vi "Actor Core.vi"(8 "error in":errorcluster, 11 "BNT_DSCXYGraph in":refnum<class "BNT_DSCXYGraph.lvclass">) -> (0 "error out":errorcluster, 3 "Actor out":refnum<class "Actor.lvclass">)   [LabVIEW 2017, in "BNT_DSCXYGraph.lvlib" / "BNT_DSCXYGraph.lvclass"]
doc: "(<B>Filename</B>: Actor Framework.lvlib:Actor.lvclass:Actor Core.vi)\n\nReceives messages to the actor, reacts to them, and initiates any error handling that may shut the actor down.\n\nDescendant classes may override this VI to append parallel tasks for the actor to complete while it handles messages. Overrides use the Call Parent Method node."
uses:
  BNT_DSCXYGraph.lvclass
  CSPP_Core/Actors/CS++BaseActor/CS++BaseActor.lvclass
  CSPP_Core/Libraries/Utilities/CS++Utilities.lvlib
  <vilib>/ActorFramework/Stop Msg/Stop Msg.lvclass
  <vilib>/ActorFramework/Actor/Actor.lvclass
  BNT_DSCXYGraph Messages/Read Decimated Traces Msg/Read Decimated Traces Msg.lvclass
  CSPP_Core/Actors/CS++GUIActor/CS++GUIActor.lvclass
  C:/User/Brand/LVP/Detlab/GemDiscProduction/Packages/CSPP_Core/Actors/CS++BaseActor/CS++BaseActor.lvclass
  C:/Program Files (x86)/National Instruments/LabVIEW 2017/vi.lib/ActorFramework/Actor/Actor.lvclass
panel:
  out "XY Graph":T1(graph)
  in  "Stop Button":bool
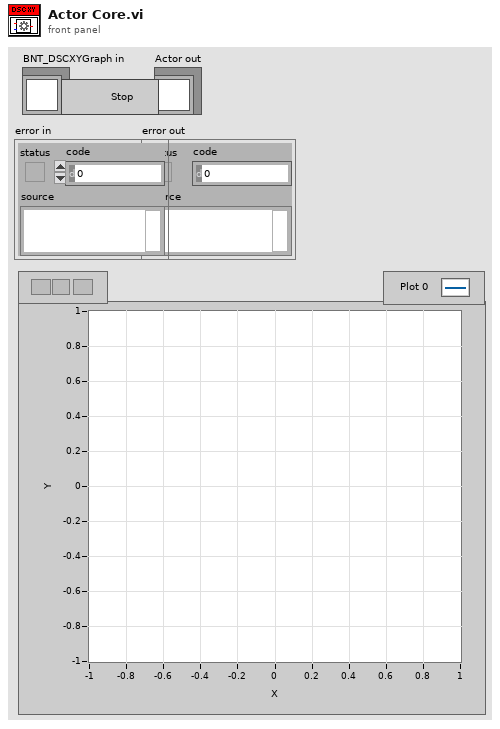
[diagram p1: front panel]
types:
  T1 = cluster{"decimated traces":dbl[], "decimated traces":dbl[]}
  T2 = enum32{"Invalid", "Standard", "Closed", "Hidden", "Minimized", "Maximized"}
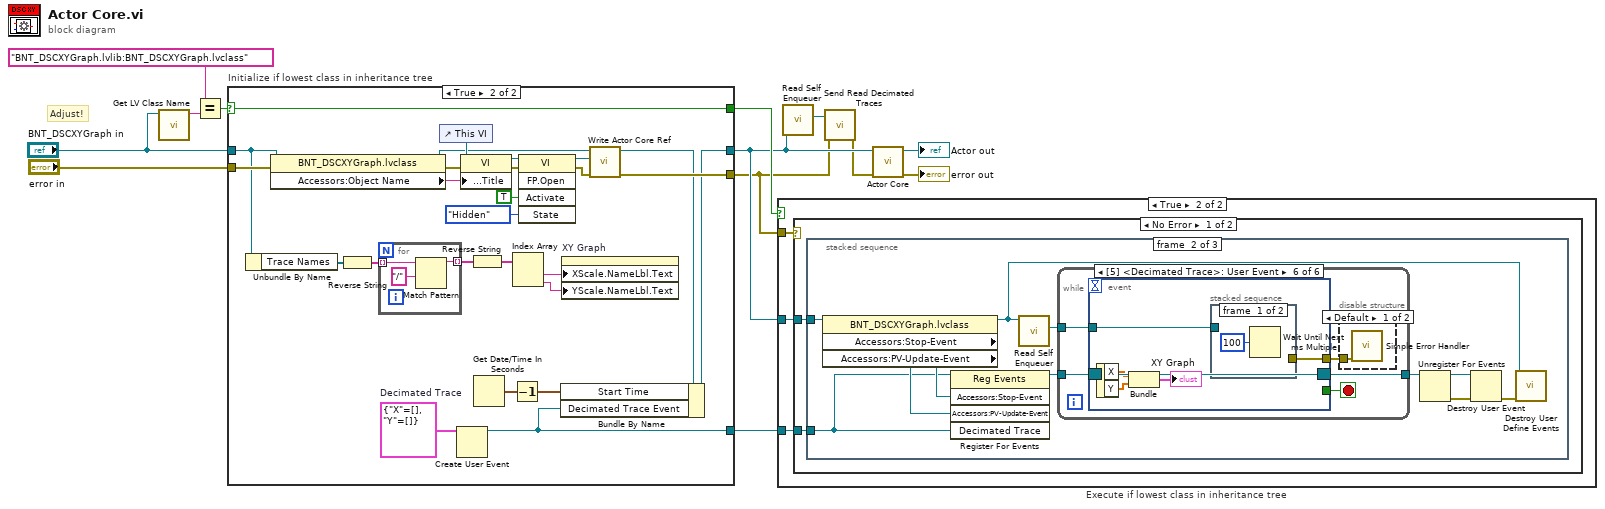
[diagram p0: block diagram]
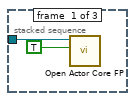
[diagram p3: hidden frame]
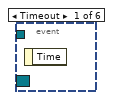
[diagram p5: hidden frame]
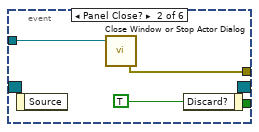
[diagram p6: hidden frame]
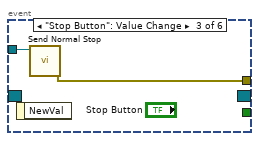
[diagram p7: hidden frame]
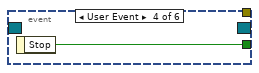
[diagram p8: hidden frame]
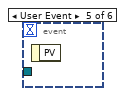
[diagram p9: hidden frame]
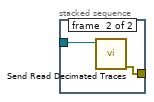
[diagram p10: hidden frame]
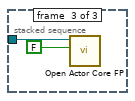
[diagram p11: hidden frame]
diagram:
  # "Adjust!"
  n1 = call <vilib>:"Get LV Class Name.vi"("object"="BNT_DSCXYGraph in") -> ("class name"=w13:string)  [unwired: 9 in, 1 out]
  n2 = Equal?(x="BNT_DSCXYGraph.lvlib:BNT_DSCXYGraph.lvclass" ("class name"), y=w13) -> (x = y?=w11:bool)
  n3 = case "Initialize if lowest class in inheritance tree" shown="True" w11 {
    selector: w11 -> [w16 w40]
    tunnel: "error in" -> [w14 w38]
    tunnel: "BNT_DSCXYGraph in" -> [w15 w29]
    tunnel: [w15 w20] -> w4
    tunnel: [w14 w36] -> w1
    tunnel: [w16 w40] -> w10
    tunnel: [_ w19] -> w5
    frame False {
    }
    frame True {
      w22 = cluster{"X":dbl[], "Y":dbl[]} {"X"=[], "Y"=[]}  # Decimated Trace
      n4 = Unbundle By Name(w29) -> ("Trace Names"=w26:refnum<k21>[])
      n5 = property class="BNT_DSCXYGraph.lvclass"(reference=w29, error in=w38) -> (reference out=w30:refnum<class "BNT_DSCXYGraph.lvclass">, error out=w32:errorcluster, "Accessors:Object Name"=w31:string)
      n6 = Reverse String(1:w26) -> (0:w28:string[])
      n7 = for {
        tunnel: w28 -> [w45] mode=indexing
        tunnel: [w43] -> w27 mode=indexing
        n8 = Match Pattern(string=w45, regular expression="/") -> (before substring=w43:string)  [unwired: 1 in, 3 out]
      }
      n9 = control-ref of="This VI"() -> (w35:refnum<vi>)
      n10 = Create User Event(user event datatype=w22) -> (user event=w19:refnum<user-event>)  [unwired: 1 in, 1 out]
      n11 = property class="VI"(reference=w35, error in=w32, "Front Panel.Title"=w31) -> (reference out=w34:refnum<vi>, error out=w33:errorcluster)
      n12 = Reverse String(1:w27) -> (0:w25:string[])
      n13 = Get Date/Time In Seconds() -> (seconds since 1Jan1904=w18:timestamp)
      n14 = Decrement(x=w18) -> (x-1=w17:timestamp)
      n15 = Index Array(array=w25) -> (element #1=w24:string, element #2=w23:string)  [unwired: 2 in]
      n16 = invoke class="VI" method="FP.Open"(reference=w34, error in=w33, "Activate"=TRUE ("Activate?"), "State"=T2."Hidden") -> (reference out=w39:refnum<vi>, error out=w37:errorcluster)  [unwired: 1 in, 3 out]
      n17 = property on="XY Graph" class="XYGraph (strict)"("XScale.NameLbl.Text"=w24, "YScale.NameLbl.Text"=w23) -> ()  [unwired: 2 in, 2 out]
      n18 = call "Write Actor Core Ref.vi"("error in (no error)"=w37, "Actor Core Ref"=w39, "CS++BaseActor in"=w30) -> ("error out"=w36:errorcluster, "CS++BaseActor out"=w21:refnum<class "BNT_DSCXYGraph.lvclass">)  [unwired: 7 in]
      n19 = Bundle By Name(cluster=w21, "Start Time"=w17, "Decimated Trace Event"=w19) -> (w20:refnum<class "BNT_DSCXYGraph.lvclass">)
    }
  }
  n20 = case "Execute if lowest class in inheritance tree" shown="True" w10 {
    tunnel: w4 -> [_ w48]
    tunnel: w1 -> [_ w47]
    tunnel: w5 -> [_ w46]
    frame False {
    }
    frame True {
      n21 = case shown="No Error" w47 {
        tunnel: w48 -> [w50 _]
        tunnel: w46 -> [w49 _]
        frame No Error {
          n22 = stacked-sequence {
            tunnel: w50 -> [w52 w62 w84]
            tunnel: w49 -> [_ w53 _]
            frame #0 {
              n23 = call "Open Actor Core FP.vi"("Open FP (F)"=TRUE, "CS++BaseActor in"=w52) -> ()  [unwired: 8 in, 2 out]
            }
            frame #1 {
              n24 = property class="BNT_DSCXYGraph.lvclass"(reference=w62) -> (reference out=w60:refnum<class "BNT_DSCXYGraph.lvclass">, "Accessors:Stop-Event"=w57:refnum<user-event>, "Accessors:PV-Update-Event"=w56:refnum<user-event>)  [unwired: 1 in, 1 out]
              n25 = register-events(w57, w56, w53) -> (reference out=w58:refnum<event-registration>)  [unwired: 2 in, 1 out]
              n26 = call <vilib>:"Read Self Enqueuer.vi"("Actor"=w60) -> ("Self Enqueuer"=w59:refnum<class "Message Enqueuer.lvclass">)  [unwired: 10 in]
              n27 = while {
                tunnel: w58 -> [w67]
                tunnel: [w65] -> w61
                tunnel: w59 -> [w63]
                stop <- w66 stop-if-true
                n28 = event shown="[5] <Decimated Trace>: User Event" {
                  selector: w67 -> [_ _ _ _ _ _]
                  dyn-events: [_ _ _ _ _ _] -> w65
                  timeout: _ -> [_ _ _ _ _ _]
                  tunnel: [_ _ _ w74 _ _] -> w66
                  tunnel: [_ w69 w73 _ _ w75] -> w64
                  tunnel: w63 -> [_ w70 w72 _ _ w76]
                  event Timeout {
                    n29 = event-data() -> ()  [unwired: 1 in, 1 out]
                  }
                  event Panel Close? {
                    n30 = event-data() -> ()  [unwired: 1 in, 1 out]
                    n31 = call "Close Window or Stop Actor Dialog.vi"("Self Enqueuer"=w70) -> ("Error Out"=w69:errorcluster)  [unwired: 2 in]
                    n32 = event-data("Discard?"=TRUE) -> ()  [unwired: 1 in, 1 out]
                  }
                  event "Stop Button": Value Change {
                    n33 = event-data() -> ()  [unwired: 1 in, 1 out]
                    n34 = call <vilib>:"Send Normal Stop.vi"("Message Enqueuer"=w72) -> ("error out"=w73:errorcluster)  [unwired: 10 in]
                  }
                  event User Event {
                    n35 = event-data() -> ("Stop"=w74:bool)  [unwired: 1 in]
                  }
                  event User Event {
                    n36 = event-data() -> ()  [unwired: 1 in, 1 out]
                  }
                  event User Event {
                    n37 = event-data() -> ("X"=w79:dbl[], "Y"=w78:dbl[])  [unwired: 1 in]
                    n38 = Bundle("X"=w79, "Y"=w78) -> (→"XY Graph":cluster{"X":dbl[], "Y":dbl[]})  [unwired: 1 in]
                    n39 = stacked-sequence {
                      tunnel: w76 -> [_ w82]
                      tunnel: [_ w81] -> w75
                      frame #0 {
                        n40 = Wait Until Next ms Multiple(millisecond multiple=u32 100) -> ()  [unwired: 1 out]
                      }
                      frame #1 {
                        n41 = call "Send Read Decimated Traces.vi"("Message Enqueuer"=w82) -> ("error out"=w81:errorcluster)  [unwired: 9 in, 1 out]
                      }
                    }
                  }
                }
                n42 = disable-structure shown="Default" {
                  disable-tunnel: w64 -> [w68 _]
                  frame condition #0 (active) {
                    n43 = call <vilib>:"Simple Error Handler.vi"("error in (no error)"=w68) -> ()  [unwired: 4 in, 5 out]
                  }
                  frame condition #1 {
                  }
                }
              }
              n44 = Unregister For Events(event registration refnum=w61) -> (error out=w55:errorcluster)  [unwired: 1 in]
              n45 = Destroy User Event(user event=w53, error in=w55) -> (error out=w54:errorcluster)
              n46 = call-dynamic "Destroy User Define Events.vi"("error in (no error)"=w54, "CS++GUIActor in"=w60) -> ()  [unwired: 8 in, 2 out]
            }
            frame #2 {
              n47 = call "Open Actor Core FP.vi"("Open FP (F)"=FALSE, "CS++BaseActor in"=w84) -> ()  [unwired: 8 in, 2 out]
            }
          }
        }
        frame Error {
        }
      }
    }
  }
  n48 = call <vilib>:"Read Self Enqueuer.vi"("Actor"=w4) -> ("Self Enqueuer"=w3:refnum<class "Message Enqueuer.lvclass">)  [unwired: 10 in]
  n49 = call "Send Read Decimated Traces.vi"("error in (no error)"=w1, "Message Enqueuer"=w3) -> ("error out"=w2:errorcluster)  [unwired: 8 in, 1 out]
  n50 = call-parent "Actor Core.vi"("error in"=w2, "CS++GUIActor in"=w4) -> ("error out"=→"error out":errorcluster, "Actor out"=→"Actor out":refnum<class "Actor.lvclass">)  [unwired: 8 in]
